vi "Message_Reconstructor - 3 SC.vi"(4 "No. Common Bits":i32=3, 6 "No. Total Bits":i32=6, 10 "Wp":u8[](array[numeric]), 11 "Wc":u8[](array[numeric])) -> (3 "W1":u8[](array[numeric]))   [LabVIEW 2022 SP3]
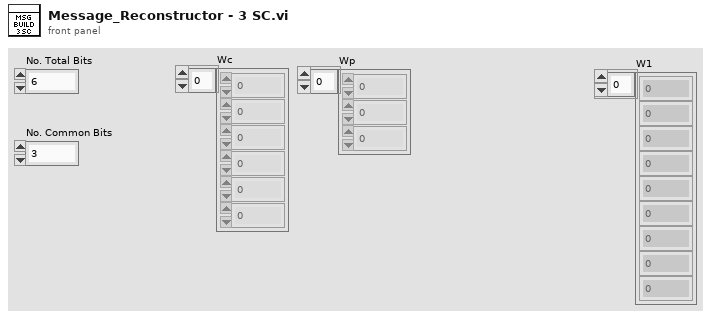
[diagram p1: front panel]
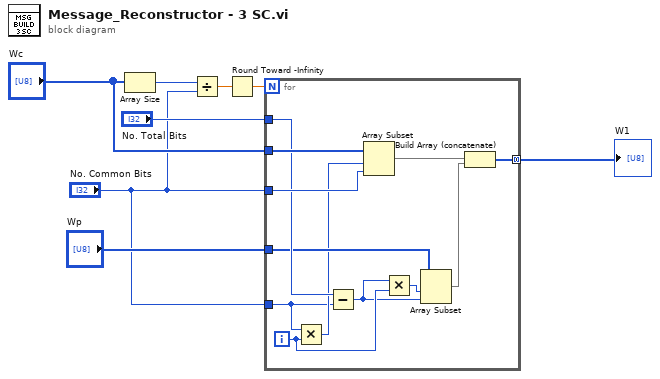
[diagram p0: block diagram]
diagram:
  n1 = Array Size(array="Wc") -> (size(s)=w8:i32)
  n2 = Divide(x=w8, y="No. Common Bits") -> (x/y=w7:dbl)
  n3 = Round Toward -Infinity(1:w7) -> (0:w6:dbl)
  n4 = for {
    N: w6 -> [_]
    tunnel: "Wc" -> [w20]
    tunnel: "No. Common Bits" -> [w12]
    tunnel: "No. Common Bits" -> [w16]
    tunnel: [w18] -> w4 mode=concatenating
    tunnel: "Wp" -> [w14]
    tunnel: "No. Total Bits" -> [w15]
    i -> [w10]
    n5 = Multiply(x=w12, y=w10) -> (x*y=w13:i32)
    n6 = Subtract(x=w15, y=w12) -> (x-y=w9:i32)
    n7 = Array Subset(array=w20, index=w13, length=w16) -> (w17:u8[])
    n8 = Multiply(x=w9, y=w10) -> (x*y=w11:i32)
    n9 = Array Subset(array=w14, index=w11, length=w9) -> (w19:u8[])
    n10 = Build Array (concatenate)(w17, w19) -> (w18:u8[])
  }
  "W1" <- w4
